vi "AudioTest.Config, Get SoundCheck Graph Definitions.vi"(11 "Config Folder":path=path "C:/MTE/Audio Test/Config") -> (0 "error out":errorcluster, 2 "Graph Names":string[](array[string]), 3 "Graph Defs":T1[](array[typedef]))   [LabVIEW 2018]
uses:
  TypeDefs/AudioTest.Graph Definitions.ctl
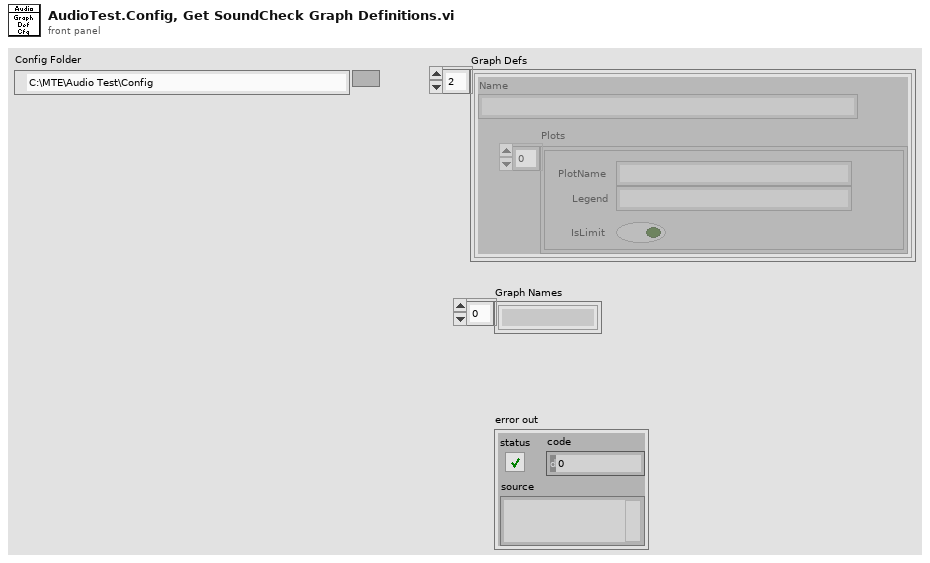
[diagram p1: front panel]
types:
  T1 = typedef "AudioTest.Graph Definitions.ctl" = cluster{"Name":string, "Plots":cluster{"PlotName":string, "Legend":string, "IsLimit":bool}[]}
  T2 = cluster{"PlotName":string, "Legend":string, "IsLimit":bool}
  T3 = cluster{"PlotName":string, "Legend":string, "IsLimit":bool}[]
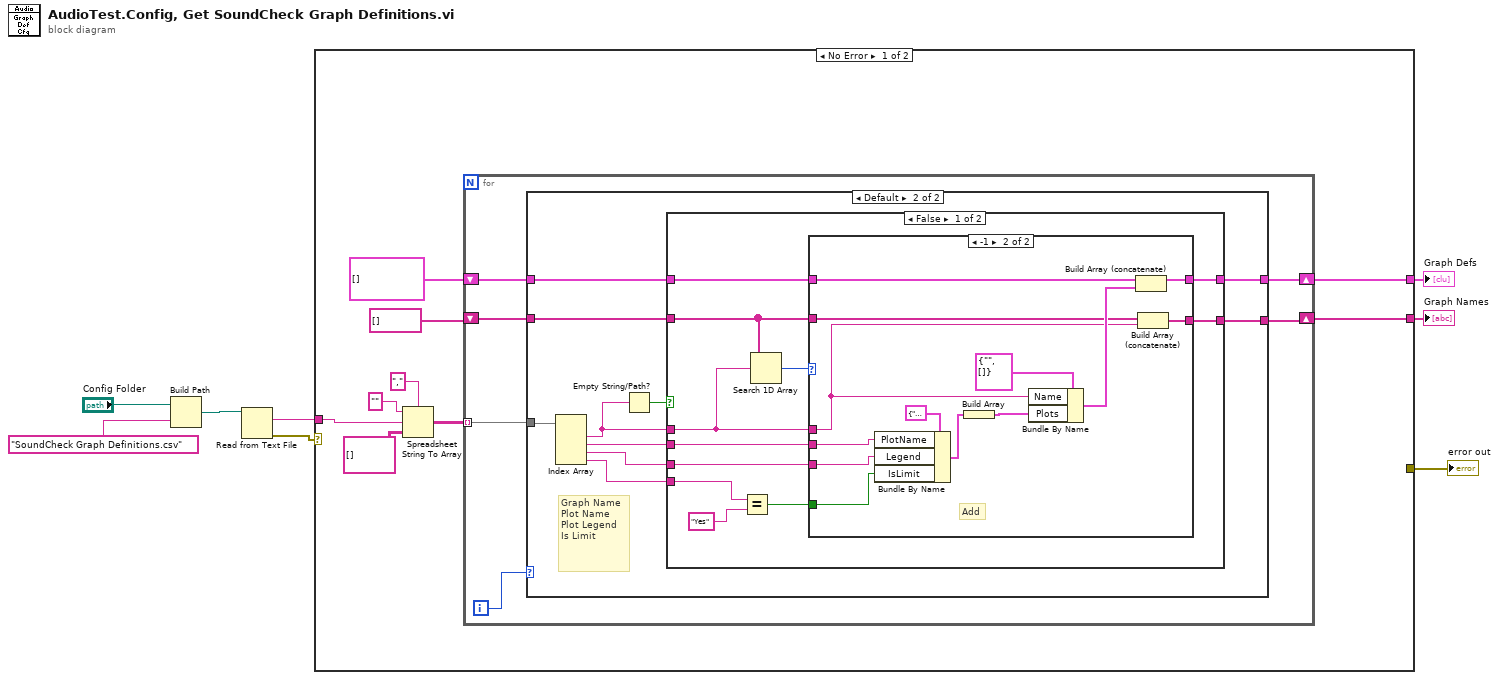
[diagram p0: block diagram]
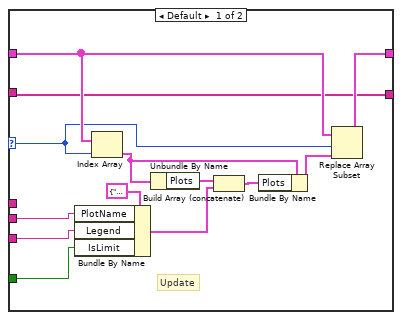
[diagram p3: hidden frame]
diagram:
  n1 = Build Path(base path="Config Folder", name or relative path="SoundCheck Graph Definitions.csv") -> (appended path=w6:path)
  n2 = Read from Text File(file (use dialog)=w6) -> (text=w5:string, error out=w4:errorcluster)  [unwired: 3 in, 2 out]
  n3 = case shown="No Error" w4 {
    selector: w4 -> [_ w75]
    tunnel: w5 -> [w17 _]
    tunnel: [w12 _] -> w2
    tunnel: [_ w75] -> w3
    tunnel: [w9 _] -> w1
    frame No Error {
      n4 = Spreadsheet String To Array(delimiter (Tab)=",", format string="", spreadsheet string=w17, array type (2D Dbl)=string[][] []) -> (array=w13:string[][])
      n5 = for {
        tunnel: w13 -> [w20] mode=indexing
        shift-right: [w21] -> w12
        shift-left: T1[] [] -> [w22]
        shift-right: [w18] -> w9
        shift-left: string[] [] -> [w19]
        i -> [w23]
        n6 = case shown="Default" w23 {
          tunnel: w22 -> [w25 w35]
          tunnel: [w25 w34] -> w21
          tunnel: w20 -> [_ w33]
          tunnel: w19 -> [w24 w27]
          tunnel: [w24 w26] -> w18
          frame 0 {
            # "Skip Heading"
          }
          frame Default {
            # "Graph Name\nPlot Name\nPlot Legend\nIs Limit"
            n7 = Index Array(array=w33) -> (element #1=w31:string, element #2=w32:string, element #3=w29:string, element #4=w28:string)  [unwired: 4 in]
            n8 = Empty String/Path?(string/path=w31) -> (empty?=w30:bool)
            n9 = case shown="False" w30 {
              tunnel: w35 -> [w45 w74]
              tunnel: [w44 w74] -> w34
              tunnel: w31 -> [w38 _]
              tunnel: w32 -> [w43 _]
              tunnel: w29 -> [w42 _]
              tunnel: w28 -> [w41 _]
              tunnel: w27 -> [w37 w73]
              tunnel: [w36 w73] -> w26
              frame False {
                n10 = Equal?(x=w41, y="Yes") -> (x = y?=w39:bool)
                n11 = Search 1D Array(1D array=w37, element=w38) -> (index of element=w46:i32)  [unwired: 1 in]
                n12 = case shown="-1" w46 {
                  selector: w46 -> [w48 _]
                  tunnel: w45 -> [w50 w72]
                  tunnel: [w51 w71] -> w44
                  tunnel: w43 -> [w56 w66]
                  tunnel: w42 -> [w55 w65]
                  tunnel: w39 -> [w54 w64]
                  tunnel: w38 -> [_ w60]
                  tunnel: w37 -> [w47 w62]
                  tunnel: [w47 w61] -> w36
                  frame Default {
                    # "Update"
                    n13 = Bundle By Name(cluster=T2 {"PlotName"="", "Legend"="", "IsLimit"=FALSE} ("Plots"), "PlotName"=w56, "Legend"=w55, "IsLimit"=w54) -> (w57:T2)
                    n14 = Index Array(array=w50, index=w48) -> (element=w53:T1)
                    n15 = Unbundle By Name(w53) -> ("Plots"=w52:T3)
                    n16 = Build Array (concatenate)(w52, w57) -> (w59:T3)
                    n17 = Bundle By Name(cluster=w53, "Plots"=w59) -> (w49:T1)
                    n18 = Replace Array Subset(array=w50, new element=w49, index=w48) -> (w51:T1[])
                  }
                  frame -1 {
                    # "Add"
                    n19 = Bundle By Name(cluster=T2 {"PlotName"="", "Legend"="", "IsLimit"=FALSE} ("Plots"), "PlotName"=w66, "Legend"=w65, "IsLimit"=w64) -> (w67:T2)
                    n20 = Build Array(w67) -> (w69:T3)
                    n21 = Bundle By Name(cluster=T1 {"Name"="", "Plots"=[]} ("Graph"), "Name"=w60, "Plots"=w69) -> (w63:T1)
                    n22 = Build Array (concatenate)(w72, w63) -> (w71:T1[])
                    n23 = Build Array (concatenate)(w62, w60) -> (w61:string[])
                  }
                }
              }
              frame True {
                # "No name - skip"
              }
            }
          }
        }
      }
    }
    frame Error {
    }
  }
  "error out" <- w3
  "Graph Defs" <- w2
  "Graph Names" <- w1
